vi "motion_create_minimum_jerk.vi"(0 "Initial Position":dbl, 5 "Final Position":dbl=1.0, 9 "Initial Time [s]":dbl, 11 "Final Time [s]":dbl=1.0, 13 "Delta Time [s]":dbl=0.001) -> (8 "Profile":cluster{"time (s)":dbl, "setpoint":dbl}[](array[cluster]) {"setpoint" format="%.2f"; "time (s)" format="%.3f"})   [LabVIEW 2015]
panel:
  out "XY Graph":cluster{"X":dbl, "Y":dbl}[](graph)
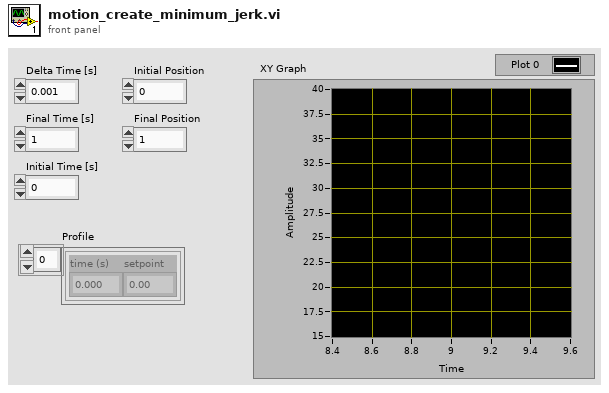
[diagram p1: front panel]
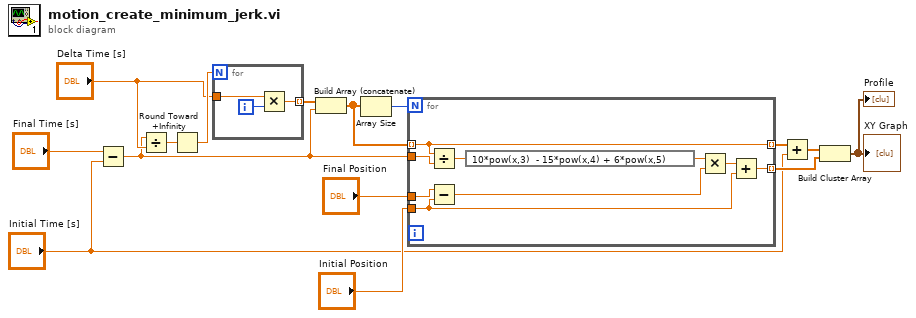
[diagram p0: block diagram]
diagram:
  n1 = Subtract(x="Final Time [s]", y="Initial Time [s]") -> (x-y=w5:dbl)
  n2 = Divide(x=w5, y="Delta Time [s]") -> (x/y=w12:dbl)
  n3 = Round Toward +Infinity(x=w12) -> (ceil(x): smallest int >= x=w11:dbl)
  n4 = for {
    N: w11 -> [_]
    tunnel: "Delta Time [s]" -> [w17]
    tunnel: [w16] -> w9 mode=indexing
    i -> [w18]
    n5 = Multiply(x=w17, y=w18) -> (x*y=w16:dbl)
  }
  n6 = Build Array (concatenate)(w9, w5) -> (w4:dbl[])
  n7 = Array Size(array=w4) -> (size(s)=w8:i32)
  n8 = for {
    N: w8 -> [_]
    tunnel: [w24] -> w15 mode=indexing
    tunnel: [w20] -> w3 mode=indexing
    tunnel: w5 -> [w23]
    tunnel: w4 -> [w20] mode=indexing
    tunnel: "Final Position" -> [w22]
    tunnel: "Initial Position" -> [w21]
    n9 = Divide(x=w20, y=w23) -> (x/y=w19:dbl)
    n10 = Subtract(x=w22, y=w21) -> (x-y=w25:dbl)
    n11 = expression code="10*pow(x,3)  - 15*pow(x,4) + 6*pow(x,5)"(w19) -> (w26:dbl)
    n12 = Multiply(x=w26, y=w25) -> (x*y=w27:dbl)
    n13 = Add(x=w27, y=w21) -> (x+y=w24:dbl)
  }
  n14 = Add(x=w3, y="Initial Time [s]") -> (x+y=w2:dbl[])
  n15 = Build Cluster Array(w2, w15) -> (→"Profile" →"XY Graph":cluster{dbl, dbl}[])
